vi "Obtain and Register Notifier.vi"(8 "error in (no error)":errorcluster, 9 "create if not found? (T)":bool=TRUE, 11 "name (unnamed)":string) -> (0 "error out":errorcluster, 1 "created new?":bool, 3 "notifier out":refnum<notifier>)   [LabVIEW 2023]
doc: "This VI obtains a new reference to a queue if it exists or creates a new queue if it does not. It also registers it in a registry which is simply an array of all queue references. The registry can be used to monitor queues and provides a single database for all queues. All queues created using this VI will be registered in volatile, global memory space.\n\nAll queues that are created by this VI are of the varient type. these VIs assume that you will be converting all queue elements to variants before enqueueing or dequeueing. To make every queue is registered, this VI must be non-reentrant."
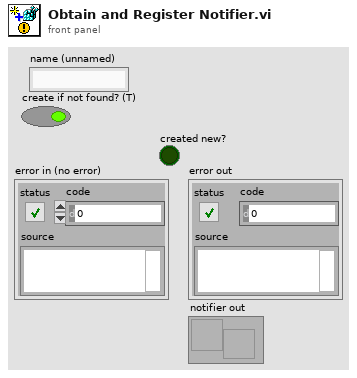
[diagram p1: front panel]
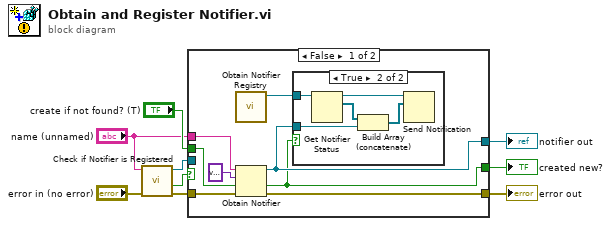
[diagram p0: block diagram]
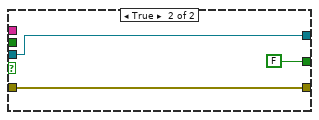
[diagram p3: hidden frame]
diagram:
  n1 = call "Check if Notifier is Registered.vi"("error in (no error)"="error in (no error)", "name (unnamed)"="name (unnamed)") -> ("error out"=w3:errorcluster, "Registered?"=w2:bool, "Registered Notifier"=w4:refnum<notifier>)  [unwired: 7 in]
  n2 = case shown="False" w2 {
    tunnel: [w12 w25] -> w6
    tunnel: w4 -> [_ w25]
    tunnel: "name (unnamed)" -> [w14 _]
    tunnel: w3 -> [w13 w23]
    tunnel: "create if not found? (T)" -> [w16 _]
    tunnel: [w11 FALSE ("created new?")] -> w8
    tunnel: [w10 w23] -> w7
    frame False {
      n3 = call "Obtain Notifier Registry.vi"() -> ("Notifier Registry"=w17:refnum<notifier>)  [unwired: 10 in, 1 out]
      n4 = Obtain Notifier(name (unnamed)=w14, notification data type=variant, create if not found? (T)=w16, error in (no error)=w13) -> (notifier out=w12:refnum<notifier>, created new?=w11:bool, error out=w10:errorcluster)
      n5 = case shown="True" w11 {
        tunnel: w12 -> [_ w22]
        tunnel: w17 -> [_ w21]
        frame False {
        }
        frame True {
          n6 = Get Notifier Status(notifier=w21) -> (notifier out=w18:refnum<notifier>, current notification=w20:refnum<notifier>[])  [unwired: 1 in, 3 out]
          n7 = Build Array (concatenate)(w20, w22) -> (w19:refnum<notifier>[])
          n8 = Send Notification(notification=w19, notifier=w18) -> ()  [unwired: 1 in, 2 out]
        }
      }
    }
    frame True {
    }
  }
  "created new?" <- w8
  "error out" <- w7
  "notifier out" <- w6
